vi "arrays.vi"() -> ()   [LabVIEW 2020]
uses:
  b2268c9c-cc86-4604-aaed-5b7206d4fd3b.vi
  226ddf1d-9ba1-49b5-92ab-96a21bddb2c0.vi
panel:
  out "Array 3":i32[](array[numeric])
  out "Array 2":bool[](array[boolean])
  out "array out 2":dbl[](array[numeric])
  out "array out":dbl[](array[numeric])
  out "index of element":i32
  in  "element 2":dbl
  out "output array 3":dbl[][](array[numeric])
  out "min index(es)":i32
  out "max index(es)":i32
  out "min value":dbl
  out "max value":dbl
  out "subarray":dbl[](array[numeric])
  out "appended array":dbl[](array[numeric])
  in  "Numeric 5":dbl
  in  "Numeric 4":dbl
  in  "Numeric 3":dbl
  in  "Numeric 2":dbl
  in  "Numeric":dbl
  out "initialized array 2":bool[](array[boolean])
  out "initialized array":dbl[](array[numeric])
  out "deleted portion":u16[](array[numeric])
  out "array w/ subset deleted":u16[](array[numeric])
  in  "Tacometro":u16(knob) scale=0.0..10.0
  in  "barra":u16(slide) scale=0.0..10.0
  out "output array 2":u16[](array[numeric])
  out "size(s)":i32
  in  "Array":u16[](array[slide]) scale=0.0..10.0
  out "element":string
  out "output array":bool[](array[boolean])
  out "dato3":dbl
  out "dato2":dbl
  out "dato1":dbl
  in  "Arreglo Double":dbl[](array[slide]) scale=0.0..100.0
  in  "Arreglo cadena":string[](array[string])
  in  "Arreglo Booleano":bool[](array[boolean])
  # "Arreglos"
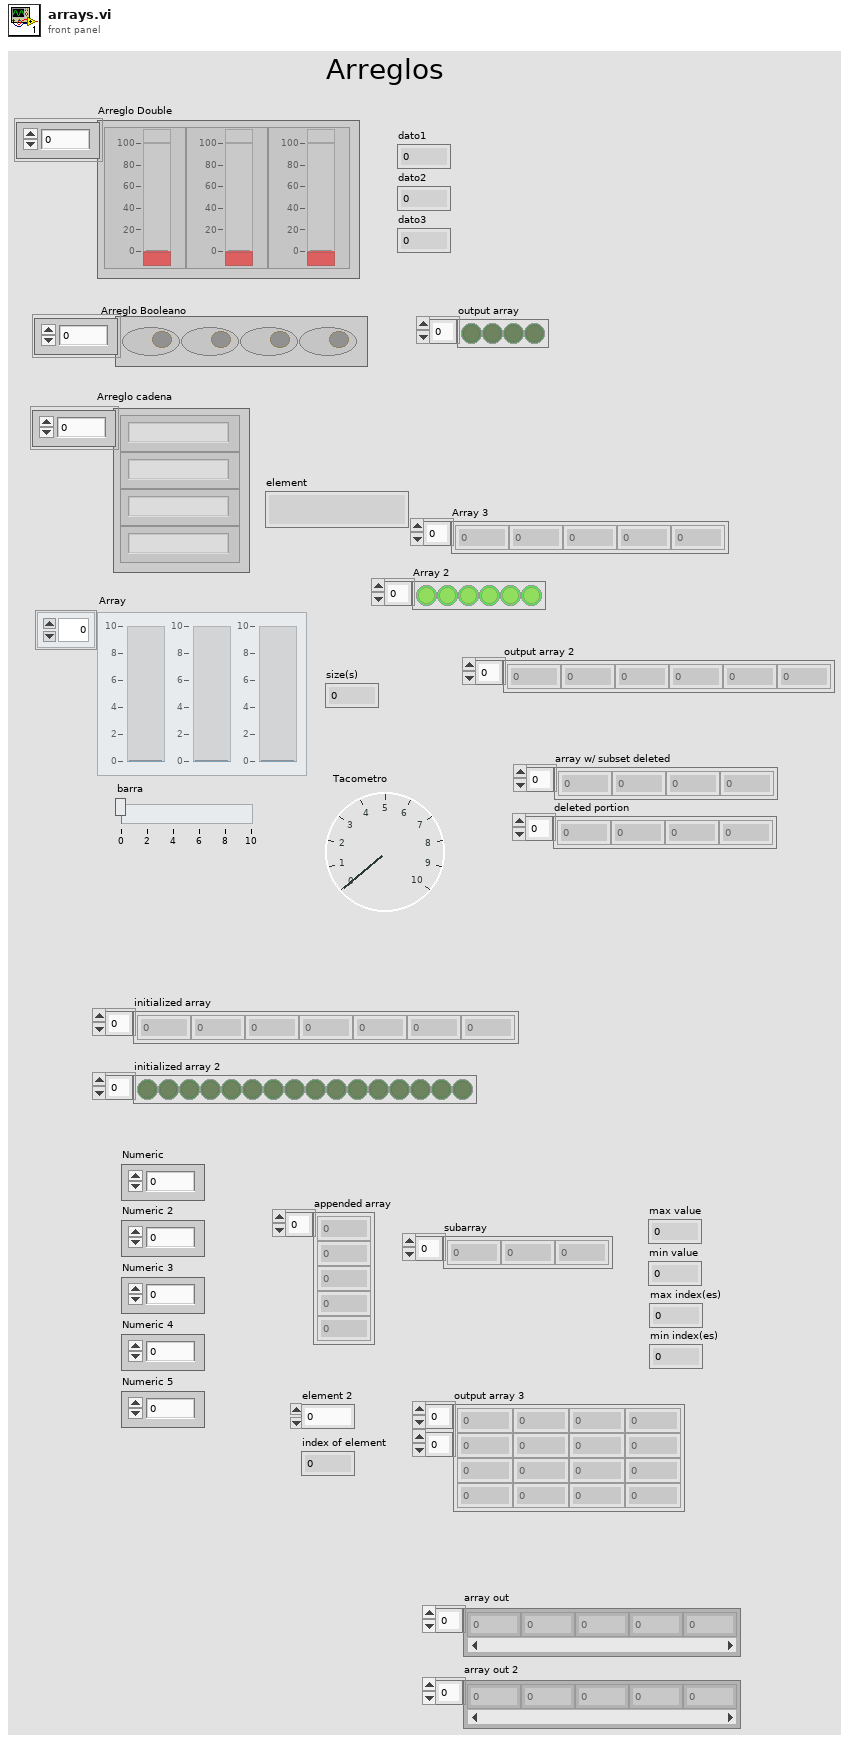
[diagram p1: front panel]
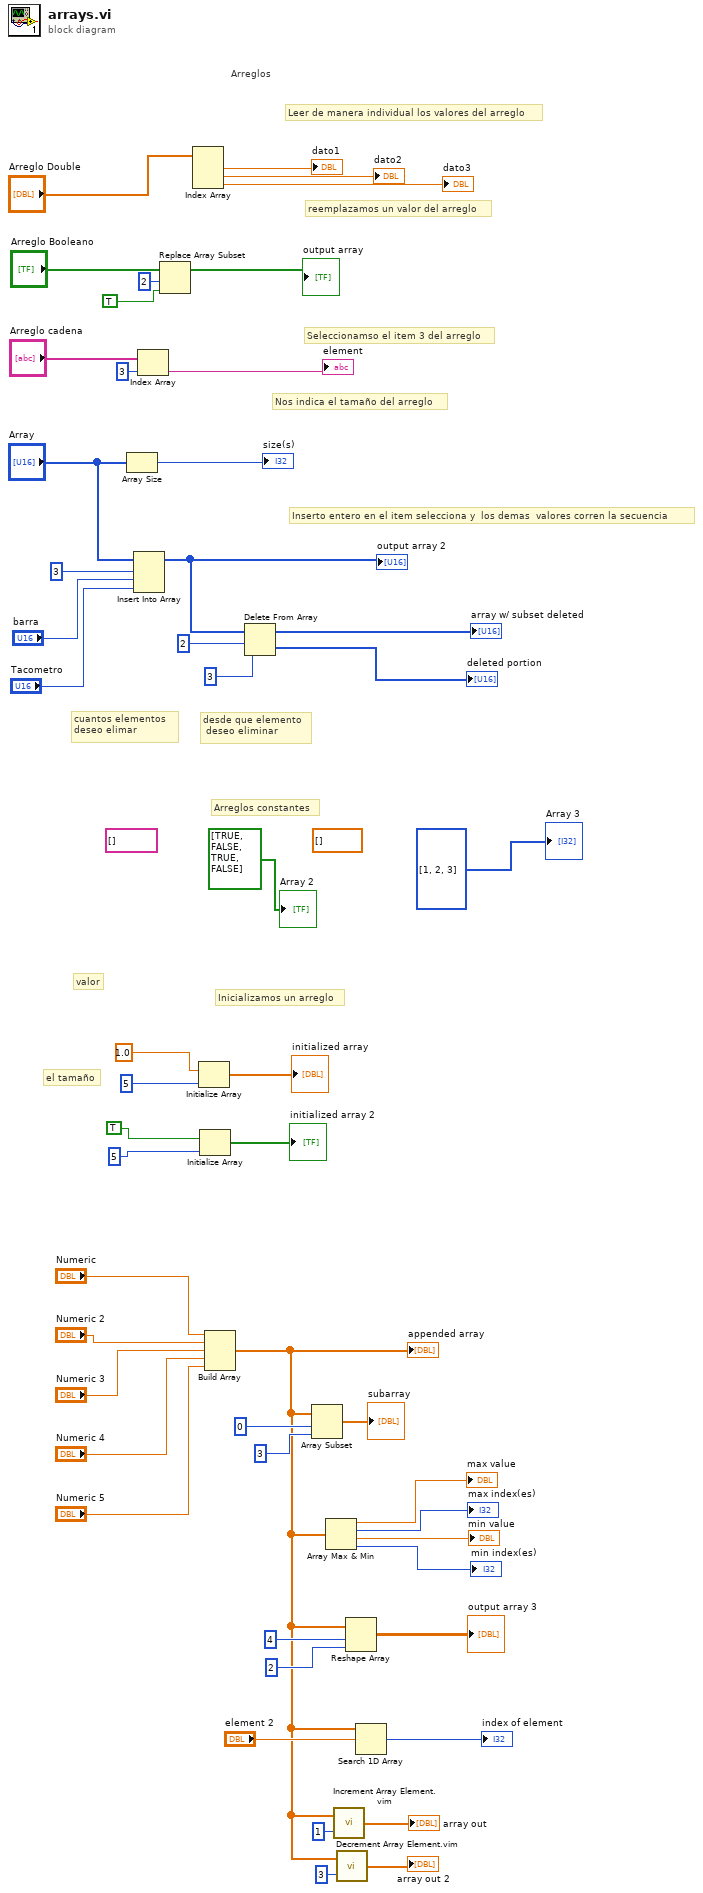
[diagram p0: block diagram]
diagram:
  (unwired) dbl[] []
  (unwired) string[] []
  # "el tamaño"
  # "valor"
  # "Inicializamos un arreglo"
  # "Arreglos constantes"
  # "desde que elemento\n deseo eliminar"
  # "cuantos elementos \ndeseo elimar"
  # "Inserto entero en el item selecciona y  los demas  valores corren la secuencia"
  # "Leer de manera individual los valores del arreglo"
  # "reemplazamos un valor del arreglo"
  # "Seleccionamso el item 3 del arreglo"
  # "Nos indica el tamaño del arreglo"
  # "Arreglos"
  n1 = Array Size(array="Array") -> (size(s)=→"size(s)":i32)
  n2 = Insert Into Array(array="Array", index=3, new element #1="barra", new element #2="Tacometro") -> (w35:u16[])
  "output array 2" <- w35
  n3 = Index Array(array="Arreglo cadena", index=3) -> (element=→"element":string)
  n4 = Replace Array Subset(array="Arreglo Booleano", new element=TRUE, index=2) -> (→"output array":bool[])
  n5 = Index Array(array="Arreglo Double") -> (element #1=→"dato1":dbl, element #2=→"dato2":dbl, element #3=→"dato3":dbl)  [unwired: 3 in]
  n6 = Initialize Array(1.0 ("element"), 5 ("dimension size")) -> (→"initialized array":dbl[])
  n7 = Initialize Array(TRUE, 5 ("dimension size")) -> (→"initialized array 2":bool[])
  n8 = Build Array("Numeric", "Numeric 2", "Numeric 3", "Numeric 4", "Numeric 5") -> (w7:dbl[])
  "appended array" <- w7
  n9 = Delete From Array(array=w35, length=2, index=3) -> (deleted portion=→"deleted portion":u16[], array with subset deleted=→"array w/ subset deleted":u16[])
  n10 = Array Subset(array=w7, index=0, length=3) -> (→"subarray":dbl[])
  n11 = Array Max & Min(array=w7) -> (max value=→"max value":dbl, max index (indices)=→"max index(es)":i32, min value=→"min value":dbl, min index (indices)=→"min index(es)":i32)
  n12 = call "Increment Array Element.vim"("index"=1, "array in"=w7) -> ("array out"=→"array out":dbl[])
  n13 = call "Decrement Array Element.vim"("index"=3, "array in"=w7) -> ("array out"=→"array out 2":dbl[])
  n14 = Reshape Array(w7, 4 ("dimension size"), 2 ("dimension size")) -> (→"output array 3":dbl[][])
  n15 = Search 1D Array(1D array=w7, element="element 2") -> (index of element=→"index of element":i32)  [unwired: 1 in]
  "Array 2" <- bool[] [TRUE, FALSE, TRUE, FALSE]
  "Array 3" <- i32[] [1, 2, 3]
